vi "Eval.MATLAB.vi"(0 "input":string, 1 "reference":refnum<k24>) -> ()   [LabVIEW 2014]
uses:
  D:/Desktop/app/LabVIEW/MLApp.dll
  MLApp.dll
panel:
  out "result":string
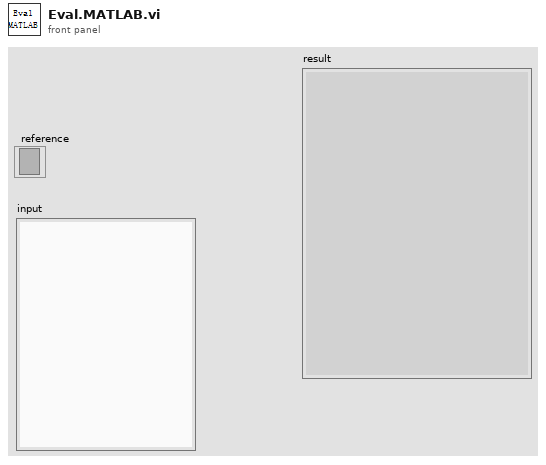
[diagram p1: front panel]
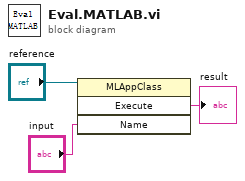
[diagram p0: block diagram]
diagram:
  n1 = invoke class="MLAppClass" method="Execute"(reference="reference", "Name"="input") -> ("Execute"=→"result":string)  [unwired: 2 in, 3 out]
